vi "SSC DCPower Wait for Event.vi"(0 "DCPower SSC in":T2[](array[typedef]), 1 "Timeout (10s)":dbl=10.0, 9 "Event":T1=1030 items=["Source Complete Event"=1030, "Measure Complete Event"=1031, "Sequence Iteration Complete Event"=1032, "Sequence Engine Done Event"=1033, "Pulse Complete Event"=1051, "Ready For Pulse Trigger Event"=1052], 11 "error in":errorcluster) -> (4 "DCPower SSC out":T2[](array[typedef]), 15 "error out":errorcluster)   [LabVIEW 2019]
doc: "This VI waits until the devices have generated the specified event."
uses:
  SSC DCPower.ctl
  <instrlib>/niDCPower/nidcpower.llb/niDCPower Wait For Event - Event.ctl
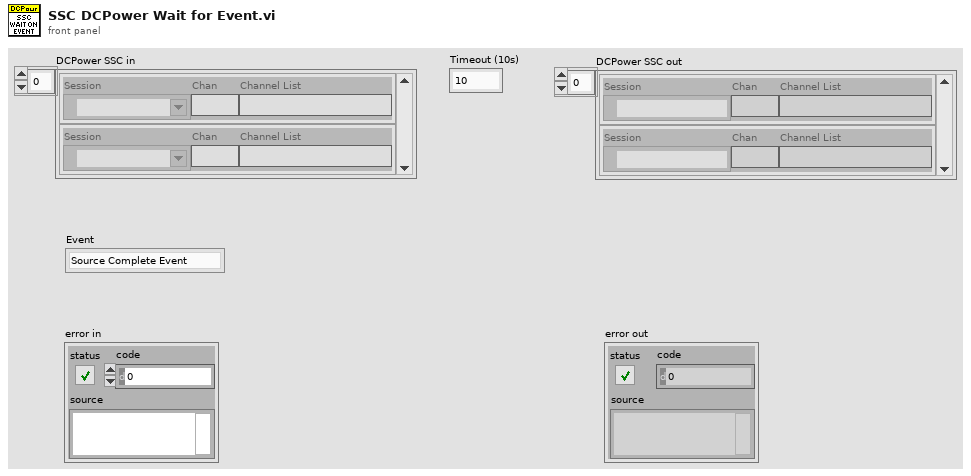
[diagram p1: front panel]
types:
  T1 = typedef "niDCPower Wait For Event - Event.ctl" = i32
  T2 = typedef "SSC DCPower.ctl" = cluster{"Session":refnum<k15>, "Chan":string, "Channel List":string}
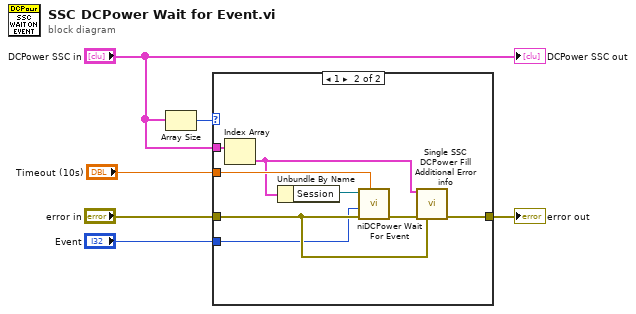
[diagram p0: block diagram]
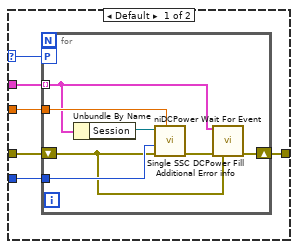
[diagram p2: hidden frame]
diagram:
  n1 = Array Size(array="DCPower SSC in") -> (size(s)=w2:i32)
  n2 = case shown="1" w2 {
    selector: w2 -> [w8 _]
    tunnel: [w12 w27] -> w6
    tunnel: "error in" -> [w11 w26]
    tunnel: "Timeout (10s)" -> [w10 w25]
    tunnel: "Event" -> [w9 w24]
    tunnel: "DCPower SSC in" -> [w7 w23]
    frame Default {
      n3 = for {
        tunnel: w7 -> [w14] mode=indexing
        workers-P: w8 -> [_]
        tunnel: w10 -> [w18]
        tunnel: w9 -> [w17]
        shift-right: [w15] -> w12
        shift-left: w11 -> [w13]
        n4 = Unbundle By Name(w14) -> ("Session"=w16:refnum<k15>)
        n5 = call <instrlib>:"niDCPower Wait For Event.vi"("timeout (sec)"=w18, "error in (no error)"=w13, "event"=w17, "instrument handle"=w16) -> ("error out"=w19:errorcluster)  [unwired: 6 in, 1 out]
        n6 = call "Single SSC DCPower Fill Additional Error info.vi"("DCPower SSC in"=w14, "error in"=w19, "previous error in"=w13) -> ("error out"=w15:errorcluster)  [unwired: 12 in]
      }
    }
    frame 1 {
      n7 = Index Array(array=w23) -> (element=w20:T2)  [unwired: 1 in]
      n8 = Unbundle By Name(w20) -> ("Session"=w21:refnum<k15>)
      n9 = call <instrlib>:"niDCPower Wait For Event.vi"("timeout (sec)"=w25, "error in (no error)"=w26, "event"=w24, "instrument handle"=w21) -> ("error out"=w22:errorcluster)  [unwired: 6 in, 1 out]
      n10 = call "Single SSC DCPower Fill Additional Error info.vi"("DCPower SSC in"=w20, "error in"=w22, "previous error in"=w26) -> ("error out"=w27:errorcluster)  [unwired: 12 in]
    }
  }
  "error out" <- w6
  "DCPower SSC out" <- "DCPower SSC in"
